vi "Measure_Resistor.vi"(8 "error in (no error)":errorcluster, 10 "Parameters":string, 11 "reference in":refnum<class "Test_Flux_Capacitor.lvclass">) -> (0 "error out":errorcluster, 2 "Result":dbl, 3 "reference out":refnum<class "Test_Flux_Capacitor.lvclass">)   [LabVIEW 2022 SP3, in "Test_Flux_Capacitor.lvlib" / "Test_Flux_Capacitor.lvclass"]
uses:
  Test_Flux_Capacitor.lvclass
  ParameterTypes/MeasureResistor.ctl
  ParameterTypes/DMM4ChanOhms.vi
  <vilib>/Analysis/baseanly.llb/Mean (DBL).vi
  <vilib>/Utility/error.llb/Trim Whitespace One-Sided.vi
  Components/SwitchBase.lvlibp/SwitchBase.lvclass
  Components/DMM_Keysight_34980A.lvlibp/DMM_Keysight_34980A.lvclass
  <vilib>/Analysis/NI_AALBase.lvlib
  <vilib>/JDP Science/JSONtext/JSONtext.lvlib
panel:
  in  "Parameter_Type":T1={"Switch"="", "Wait (msec)"=0, "Scale"=0.0, "DMM_4W_Ohms"={"Range"=enum."Auto", "Resolution"=enum."Default", "Samples"=1, "dt (s)"=0.0, "Timeout (s)"=10000.0}}
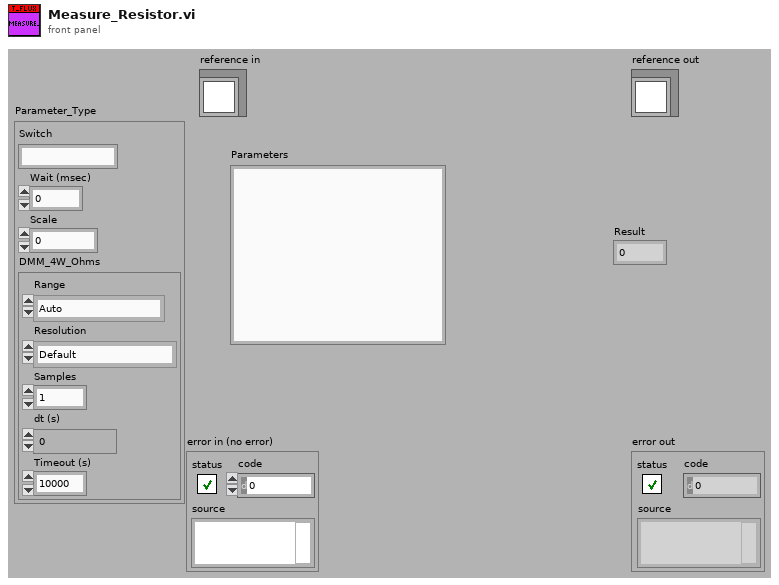
[diagram p1: front panel]
types:
  T1 = typedef "Test_Flux_Capacitor.lvlib/Test_Flux_Capacitor.lvclass/MeasureResistor.ctl" = cluster{"Switch":string, "Wait (msec)":u32, "Scale":dbl, "DMM_4W_Ohms":T2}
  T2 = typedef "Test_Flux_Capacitor.lvlib/Test_Flux_Capacitor.lvclass/DMM4ChanOhms.vi" = cluster{"Range":enum16{"100 Ohm", "1 kOhm", "10 kOhm", "100 kOhm", "1 MOhm", "10 MOhm", "100 MOhm", "Auto", "Minimum", "Maximum"}, "Resolution":enum16{"4 1/2", "5 1/2", "6 1/2", "Least", "Highest", "Default"}, "Samples":u32, "dt (s)":dbl, "Timeout (s)":dbl}
  T3 = typedef "Test_Flux_Capacitor.lvlib/Test_Flux_Capacitor.lvclass/ObjectAttributes.ctl" = cluster{"Config":T4, "DMM":refnum<class "DMM_Keysight_34980A.lvclass">, "LCR":refnum<class "LCR_BK891.lvclass">, "PSU":refnum<class "PSU_Base.lvclass">, "Switch_Manager":refnum<class "SwitchBase.lvclass">, "FRAM":string, "Flux_Capacitor":refnum<class "Flux_Capacitor.lvclass">, "Frequency_Counter":refnum<class "Frequency_Counter_Base.lvclass">, "JTAG":refnum<class "JTAG_Base.lvclass">}
  T4 = typedef "Test_Flux_Capacitor.lvlib/Test_Flux_Capacitor.lvclass/Config.ctl" = cluster{"default":string}
  T5 = enum16{"100 Ohm", "1 kOhm", "10 kOhm", "100 kOhm", "1 MOhm", "10 MOhm", "100 MOhm", "Auto", "Minimum", "Maximum"}
  T6 = enum16{"4 1/2", "5 1/2", "6 1/2", "Least", "Highest", "Default"}
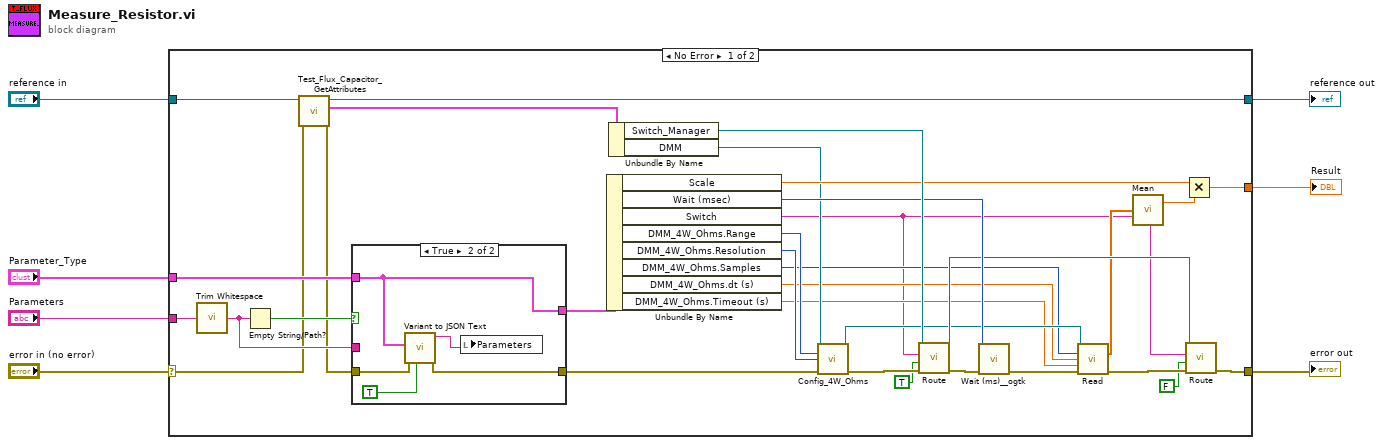
[diagram p0: block diagram]
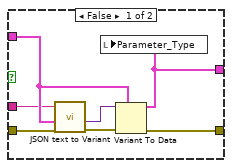
[diagram p2: hidden frame]
diagram:
  n1 = case shown="No Error" "error in (no error)" {
    selector: "error in (no error)" -> [w10 w54]
    tunnel: [w37 w54] -> w6
    tunnel: [w21 w53] -> w4
    tunnel: "reference in" -> [w23 w53]
    tunnel: "Parameters" -> [w19 _]
    tunnel: "Parameter_Type" -> [w20 _]
    tunnel: [w34 _] -> w1
    frame No Error {
      n2 = call <vilib>:"Trim Whitespace.vi"("string"=w19) -> ("trimmed string"=w26:string)  [unwired: 1 in]
      n3 = Empty String/Path?(string/path=w26) -> (empty?=w25:bool)
      n4 = call "Test_Flux_Capacitor_GetAttributes.vi"("error in (no error)"=w10, "reference in"=w23) -> ("error out"=w9:errorcluster, "Data"=w22:T3, "reference out"=w21:refnum<class "Test_Flux_Capacitor.lvclass">)  [unwired: 6 in, 1 out]
      n5 = case shown="True" w25 {
        tunnel: w9 -> [w45 w52]
        tunnel: w20 -> [w43 w49]
        tunnel: [w47 w51] -> w24
        tunnel: [w46 w49] -> w18
        tunnel: w26 -> [w42 _]
        frame False {
          n6 = call <vilib>:"JSON text to Variant.vi"("error in (no error)"=w45, "Data Type"=w43, "JSON"=w42) -> ("error out"=w44:errorcluster, "Variant out"=w41:variant)  [unwired: 7 in]
          n7 = Variant To Data(error in=w44, type=w43, Variant=w41) -> (data=w46:T1, error out=w47:errorcluster)
          n8 = local write "Parameter_Type"(w46) -> ()
        }
        frame True {
          n9 = call <vilib>:"Variant to JSON Text.vi"("Pretty Print?"=TRUE ("Enums As String (F)"), "error in (no error)"=w52, "Variant"=w49) -> ("error out"=w51:errorcluster, "<JSON>"=w48:string)  [unwired: 6 in, 1 out]
          n10 = local write "Parameters"(w48) -> ()
        }
      }
      n11 = Unbundle By Name(w18) -> ("Scale"=w35:dbl, "Wait (msec)"=w38:u32, "Switch"=w8:string, "DMM_4W_Ohms.Range"=w32:T5, "DMM_4W_Ohms.Resolution"=w33:T6, "DMM_4W_Ohms.Samples"=w17:u32, "DMM_4W_Ohms.dt (s)"=w16:dbl, "DMM_4W_Ohms.Timeout (s)"=w15:dbl)
      n12 = Unbundle By Name(w22) -> ("Switch_Manager"=w40:refnum<class "SwitchBase.lvclass">, "DMM"=w31:refnum<class "DMM_Keysight_34980A.lvclass">)
      n13 = call-dynamic "Config_4W_Ohms.vi"("reference in"=w31, "Range (7:Auto)"=w32, "Resolution (5:Default)"=w33, "error in (no error)"=w24) -> ("reference in"=w27:refnum<class "DMM_Keysight_34980A.lvclass">, "error out"=w30:errorcluster)  [unwired: 10 in]
      n14 = call-dynamic "Route.vi"("error in (no error)"=w30, "Connect"=TRUE, "channel 1"=w8, "reference in"=w40) -> ("error out"=w39:errorcluster, "reference in"=w36:refnum<class "SwitchBase.lvclass">)  [unwired: 6 in]
      n15 = call <userlib>:"Wait (ms)__ogtk.vi"("error in (no error)"=w39, "milliseconds to wait"=w38) -> ("error out"=w29:errorcluster)  [unwired: 8 in, 1 out]
      n16 = call-dynamic "Read.vi"("reference in"=w27, "Samples"=w17, "dt"=w16, "Timeout (10 s)"=w15, "error in (no error)"=w29) -> ("Measurement"=w14:dbl[], "error out"=w28:errorcluster)  [unwired: 7 in, 2 out]
      n17 = call-poly <vilib>:"Mean.vi"("X"=w14) -> ("mean"=w13:dbl)  [unwired: 1 out]
      n18 = Multiply(x=w35, y=w13) -> (x*y=w34:dbl)
      n19 = call-dynamic "Route.vi"("error in (no error)"=w28, "Connect"=FALSE, "channel 1"=w8, "reference in"=w36) -> ("error out"=w37:errorcluster)  [unwired: 6 in, 1 out]
    }
    frame Error {
    }
  }
  "Result" <- w1
  "error out" <- w6
  "reference out" <- w4
